vi "emi_Rad to Deg.vi"(7 "Rad":dbl) -> (8 "Deg":dbl)   [LabVIEW 2011]
doc: "Convert a double containgng an angle in radiance, to an angle in degrees."
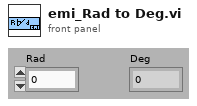
[diagram p1: front panel]
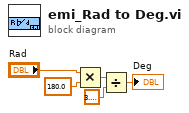
[diagram p0: block diagram]
diagram:
  n1 = Multiply(x="Rad", y=180.0) -> (x*y=w5:dbl)
  n2 = Divide(x=w5, y=3.141592653589793) -> (x/y=→"Deg":dbl)
